vi "StringParser.vi"() -> ()   [LabVIEW 2014]
panel:
  out "array":string[](array[string])
  in  "String":string
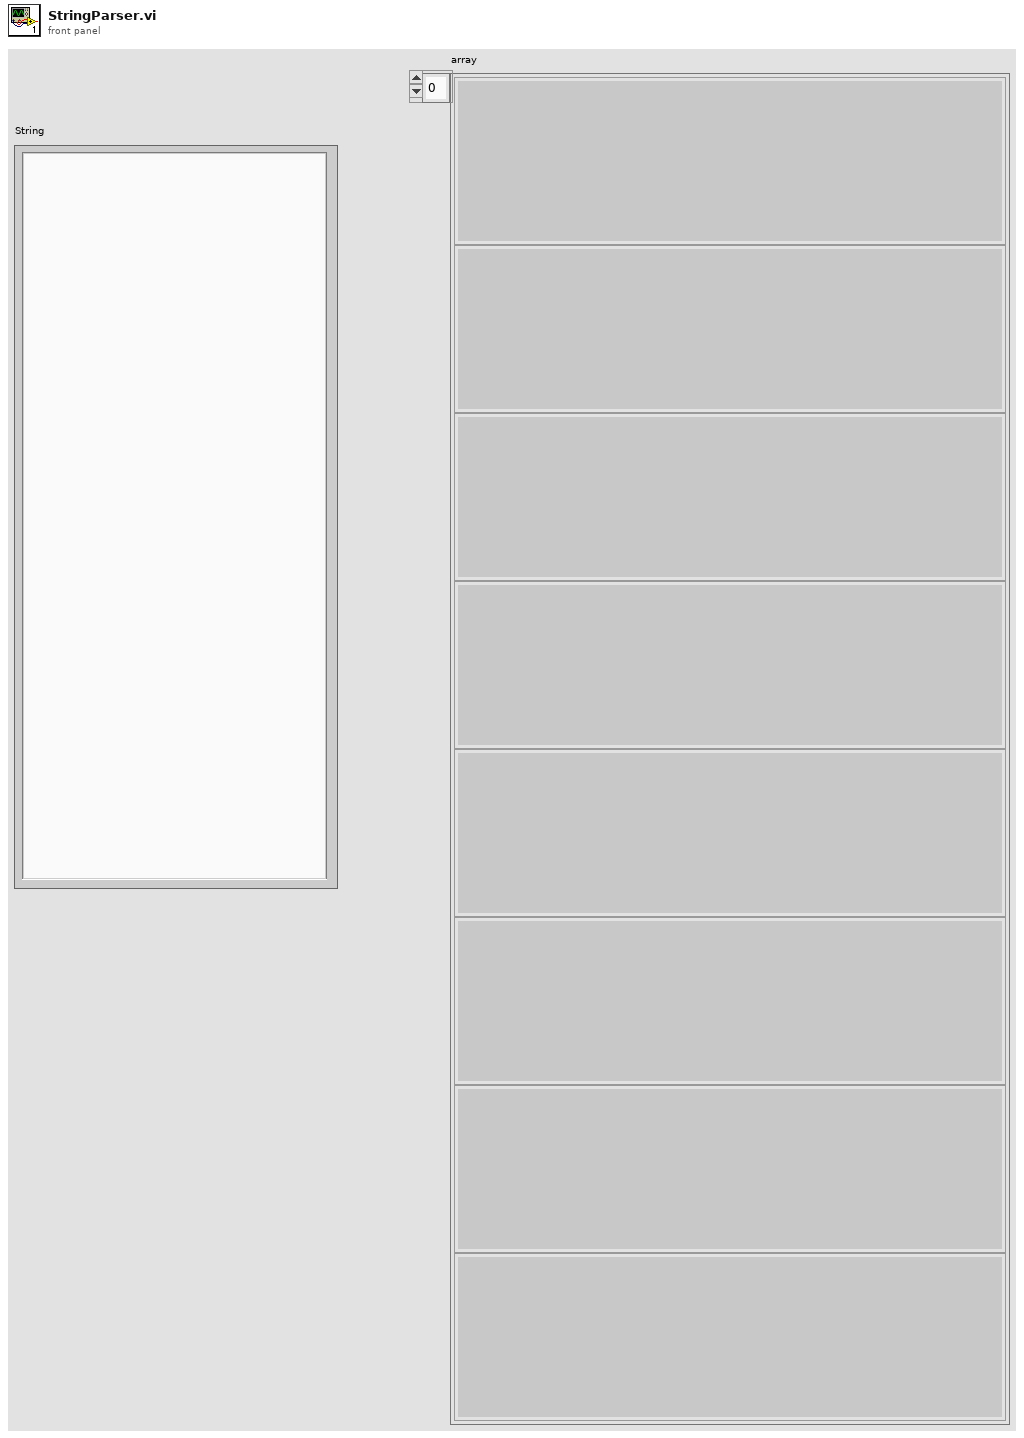
[diagram p1: front panel]
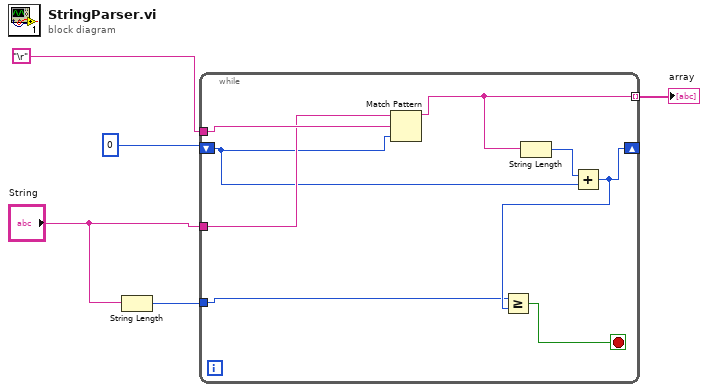
[diagram p0: block diagram]
diagram:
  n1 = String Length(string="String") -> (length=w1:i32)
  n2 = while {
    tunnel: "\r" -> [w13]
    tunnel: [w11] -> w5 mode=indexing
    tunnel: "String" -> [w12]
    shift-right: [w8] -> _
    shift-left: 0 -> [w9]
    tunnel: w1 -> [w7]
    stop <- w6 stop-if-true
    n3 = Match Pattern(string=w12, regular expression=w13, offset (0)=w9) -> (before substring=w11:string)  [unwired: 3 out]
    n4 = String Length(string=w11) -> (length=w10:i32)
    n5 = Add(x=w10, y=w9) -> (x+y=w8:i32)
    n6 = Greater Or Equal?(x=w7, y=w8) -> (x >= y?=w6:bool)
  }
  "array" <- w5
